vi "IMU.vi"() -> (0 "IMU error out":errorcluster)   [LabVIEW 2016]
panel:
  in  "stop?":bool
  in  "IMU error in":errorcluster
  in  "IMU Baud rate":u32(ring)=9600 items=["Auto Connect"=0, "300"=300, "600"=600, "1200"=1200, "2400"=2400, "4800"=4800, "9600"=9600, "19200"=19200, "38400"=38400, "57600"=57600, "115200"=115200]
  out "IMU port out":refnum<visa-resource-name>
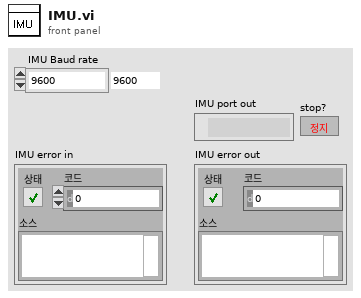
[diagram p1: front panel]
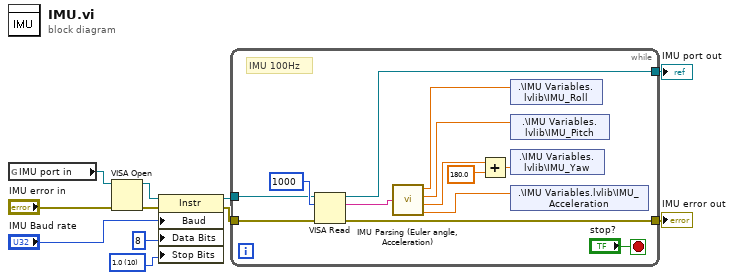
[diagram p0: block diagram]
diagram:
  w9 = u16 10 items=["1.0"=10, "1.5"=15, "2.0"=20] ("Serial Settings:Stop Bits")
  n1 = global read "[GV]_IMU Port NUM.vi" "IMU port in"() -> (w1:refnum<visa-resource-name>)
  n2 = VISA Open(error in (no error)="IMU error in", VISA resource name=w1) -> (VISA resource name=w8:refnum<visa-resource-name>, error out=w6:errorcluster)  [unwired: 3 in]
  n3 = property class="Instr"(reference=w8, error in=w6, "Baud"="IMU Baud rate", "Data Bits"=u16 8 ("Serial Settings:Data Bits"), "Stop Bits"=w9) -> (reference out=w4:refnum<visa-resource-name>, error out=w3:errorcluster)
  n4 = while {
    tunnel: w4 -> [w23]
    tunnel: w3 -> [w22]
    tunnel: [w21] -> w2
    tunnel: [w20] -> w11
    stop <- "stop?" stop-if-true
    # "IMU 100Hz"
    n5 = VISA Read(VISA resource name=w23, byte count=u32 1000 ("바이트 카운트"), error in (no error)=w22) -> (VISA resource name out=w20:refnum<visa-resource-name>, read buffer=w19:string, error out=w21:errorcluster)  [unwired: 1 out]
    n6 = call "IMU Parsing (Euler angle, Acceleration).vi"("IMU Data"=w19) -> ("IMU_Roll"=w14:dbl, "IMU_Pitch"=w16:dbl, "IMU_Yaw"=w17:dbl, "IMU Raw ax"=w13:dbl)  [unwired: 4 in]
    n7 = Add(x=w17, y=180.0) -> (x+y=w15:dbl)
    n8 = shared-variable ".\\IMU Variables.lvlib\\IMU_Roll"(w14) -> ()  [unwired: 1 in, 1 out]
    n9 = shared-variable ".\\IMU Variables.lvlib\\IMU_Pitch"(w16) -> ()  [unwired: 1 in, 1 out]
    n10 = shared-variable ".\\IMU Variables.lvlib\\IMU_Yaw"(w15) -> ()  [unwired: 1 in, 1 out]
    n11 = shared-variable ".\\IMU Variables.lvlib\\IMU_Acceleration"(w13) -> ()  [unwired: 1 in, 1 out]
  }
  "IMU port out" <- w11
  "IMU error out" <- w2
